vi "Actor Core.vi"(8 "error in":errorcluster, 11 "CS++GoBangServer in":refnum<class "CS++GoBangServer.lvclass">) -> (0 "error out":errorcluster, 3 "Actor out":refnum<class "Actor.lvclass">)   [LabVIEW 2014, in "GoBang.lvlib" / "CS++GoBangServer.lvclass"]
doc: "(<B>Filename</B>: Actor Framework.lvlib:Actor.lvclass:Actor Core.vi)\n\nReceives messages to the actor, reacts to them, and initiates any error handling that may shut the actor down.\n\nDescendant classes may override this VI to append parallel tasks for the actor to complete while it handles messages. Overrides use the Call Parent Method node."
uses:
  CS++GoBangServer.lvclass
  CSPP_Core/Actors/CS++BaseActor/CS++BaseActor.lvclass
  CSPP_Core/Actors/CS++SVMonitor/CS++SVMonitor.lvclass
  CSPP_Core/Actors/CS++PVMonitor Messages/Register PVs Msg/Register PVs Msg.lvclass
  CS++GoBangServer Messages/JoinGame Msg/JoinGame Msg.lvclass
  CS++GoBangServer Messages/Analyse Board Msg/Analyse Board Msg.lvclass
  CSPP_Core/Classes/CS++ProcessVariables/SVConnection/SVConnection.lvclass
  CSPP_Core/Classes/CS++ProcessVariables/PVConnection/PVConnection.lvclass
  CSPP_Core/Classes/CS++ProcessVariables/ProcessVariable/PV.lvclass
  <vilib>/ActorFramework/Actor/Actor.lvclass
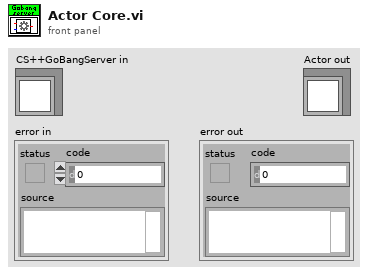
[diagram p1: front panel]
types:
  T1 = enum32{"Invalid", "Standard", "Closed", "Hidden", "Minimized", "Maximized"}
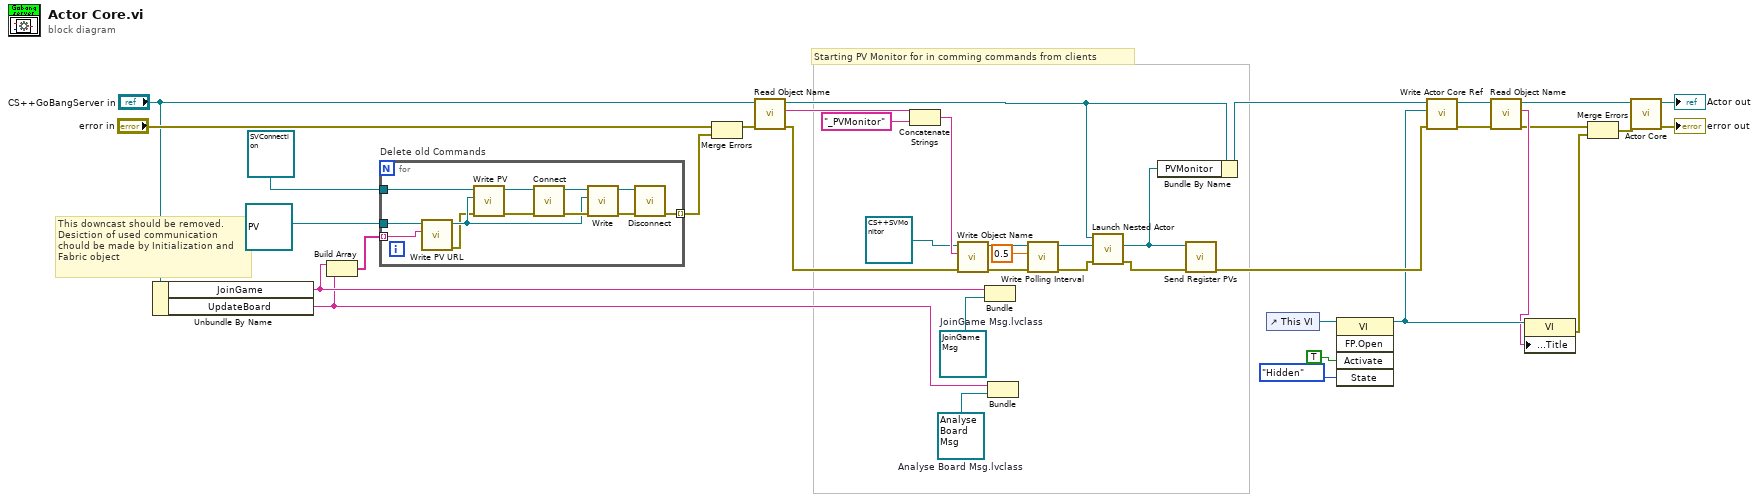
[diagram p0: block diagram]
diagram:
  w31 = refnum<class "Analyse Board Msg.lvclass"> refnum  # Analyse Board Msg.lvclass
  w32 = refnum<class "JoinGame Msg.lvclass"> refnum  # JoinGame Msg.lvclass
  # "Starting PV Monitor for in comming commands from clients"
  # "This downcast should be removed.\nDesiction of used communication \nchould be made by Initialization and\nFabric object"
  n1 = Unbundle By Name("CS++GoBangServer in") -> ("JoinGame"=w13:string, "UpdateBoard"=w12:string)
  n2 = Build Array(w13, w12) -> (w11:string[])
  n3 = for "Delete old Commands" {
    tunnel: refnum<class "SVConnection.lvclass"> refnum ("CS++ProcessVariables.lvlib:SVConnection.lvclass") -> [w44]
    tunnel: refnum<class "PV.lvclass"> refnum ("CS++ProcessVariables.lvlib:PV.lvclass") -> [w45]
    tunnel: [w47] -> w14 mode=indexing
    tunnel: w11 -> [w46] mode=indexing
    n4 = call "Write PV URL.vi"("PV URL"=w46, "PV in"=w45) -> ("error out"=w40:errorcluster, "PV out"=w43:refnum<class "PV.lvclass">)  [unwired: 8 in]
    n5 = call "Write PV.vi"("error in (no error)"=w40, "PV"=w43, "PVConnection in"=w44) -> ("error out"=w41:errorcluster, "PVConnection out"=w42:refnum<class "SVConnection.lvclass">)  [unwired: 7 in]
    n6 = call "Connect.vi"("error in (no error)"=w41, "PVConnection in"=w42) -> ("error out"=w49:errorcluster, "PVConnection out"=w51:refnum<class "SVConnection.lvclass">)  [unwired: 8 in]
    n7 = call "Write.vi"("error in (no error)"=w49, "PV"=w43, "PVConnection in"=w51) -> ("error out"=w48:errorcluster, "PVConnection out"=w50:refnum<class "SVConnection.lvclass">)  [unwired: 7 in]
    n8 = call "Disconnect.vi"("error in (no error)"=w48, "PVConnection in"=w50) -> ("error out"=w47:errorcluster)  [unwired: 8 in, 1 out]
  }
  n9 = Merge Errors("error in", w14) -> (w15:errorcluster)
  n10 = call "Read Object Name.vi"("error in (no error)"=w15, "CS++BaseActor in"="CS++GoBangServer in") -> ("error out"=w30:errorcluster, "Object Name"=w33:string, "CS++BaseActor out"=w5:refnum<class "CS++GoBangServer.lvclass">)  [unwired: 7 in]
  n11 = Concatenate Strings(w33, "_PVMonitor" ("Object Name")) -> (w36:string)
  n12 = call "Write Object Name.vi"("error in (no error)"=w30, "Object Name"=w36, "CS++BaseActor in"=refnum<class "CS++SVMonitor.lvclass"> refnum ("CS++SVMonitor.lvlib:CS++SVMonitor.lvclass")) -> ("error out"=w9:errorcluster, "CS++BaseActor out"=w10:refnum<class "CS++SVMonitor.lvclass">)  [unwired: 7 in]
  n13 = Bundle("JoinGame"=w13, "JoinGame Msg.lvclass"=w32) -> ()  [unwired: 1 in, 1 out]
  n14 = Bundle("UpdateBoard"=w12, "Analyse Board Msg.lvclass"=w31) -> ()  [unwired: 1 in, 1 out]
  n15 = call "Write Polling Interval.vi"("error in (no error)"=w9, "Polling Interval"=dbl[unit] 0.5 ("Interval"), "CS++BaseActor in"=w10) -> ("error out"=w3:errorcluster, "CS++BaseActor out"=w1:refnum<class "CS++SVMonitor.lvclass">)  [unwired: 7 in]
  n16 = call <vilib>:"Launch Nested Actor.vi"("error in (no error)"=w3, "Nested Actor"=w1, "Caller Actor in"=w5) -> ("error out"=w2:errorcluster, "Nested Actor's Enqueuer"=w4:refnum<class "Message Enqueuer.lvclass">)  [unwired: 6 in, 1 out]
  n17 = Bundle By Name(cluster=w5, "PVMonitor"=w4) -> (w29:refnum<class "CS++GoBangServer.lvclass">)
  n18 = call "Send Register PVs.vi"("error in (no error)"=w2, "Message Enqueuer"=w4) -> ("error out"=w28:errorcluster)  [unwired: 8 in, 1 out]
  n19 = control-ref of="This VI"() -> (w25:refnum<vi>)
  n20 = invoke class="VI" method="FP.Open"(reference=w25, "Activate"=TRUE ("Activate?"), "State"=T1."Hidden") -> (reference out=w22:refnum<vi>)  [unwired: 2 in, 4 out]
  n21 = call "Write Actor Core Ref.vi"("error in (no error)"=w28, "Actor Core Ref"=w22, "CS++BaseActor in"=w29) -> ("error out"=w23:errorcluster, "CS++BaseActor out"=w24:refnum<class "CS++GoBangServer.lvclass">)  [unwired: 7 in]
  n22 = call "Read Object Name.vi"("error in (no error)"=w23, "CS++BaseActor in"=w24) -> ("error out"=w18:errorcluster, "Object Name"=w21:string, "CS++BaseActor out"=w19:refnum<class "CS++GoBangServer.lvclass">)  [unwired: 7 in]
  n23 = property class="VI"(reference=w22, "Front Panel.Title"=w21) -> (error out=w20:errorcluster)  [unwired: 1 in, 1 out]
  n24 = Merge Errors(w18, w20) -> (w17:errorcluster)
  n25 = call-parent "Actor Core.vi"("error in"=w17, "CS++BaseActor in"=w19) -> ("error out"=→"error out":errorcluster, "Actor out"=→"Actor out":refnum<class "Actor.lvclass">)  [unwired: 8 in]
